vi "TSM SSC Fgen Pins to Sessions.vi"(0 "TSM context in":T3, 5 "Pins":string[](array[string]), 7 "Site Numbers":i32[](array[numeric]), 11 "error in":errorcluster) -> (4 "TSM FGEN":T1, 15 "error out":errorcluster)   [LabVIEW 2020]
doc: "Populates the TSM SSC Fgen cluster for the specified pin(s) and pin group(s)."
uses:
  <vilib>/NI_TestStand_SemiconductorModule/NI_TestStand_Semiconductor_Module.lvlibp/PinMap/General/SemiconductorModuleContext.ctl
  TSM SSC Fgen.ctl
  <vilib>/NI_TestStand_SemiconductorModule/NI_TestStand_Semiconductor_Module.lvlibp/PinMap/PinQueryContext/MultiplePinMultipleSessionQueryContext/MultiplePinMultipleSessionQueryContext.lvclass
  C:/Program Files/National Instruments/LabVIEW 2020/vi.lib/NI_TestStand_SemiconductorModule/NI_TestStand_Semiconductor_Module.lvlibp/PinMap/PinQueryContext/PinQueryContext.lvclass
  SSC Fgen.ctl
  <vilib>/NI_TestStand_SemiconductorModule/NI_TestStand_Semiconductor_Module.lvlibp/PinMap/FGEN/PinsToNIFGenSessions.vi
  <vilib>/NI_TestStand_SemiconductorModule/NI_TestStand_Semiconductor_Module.lvlibp
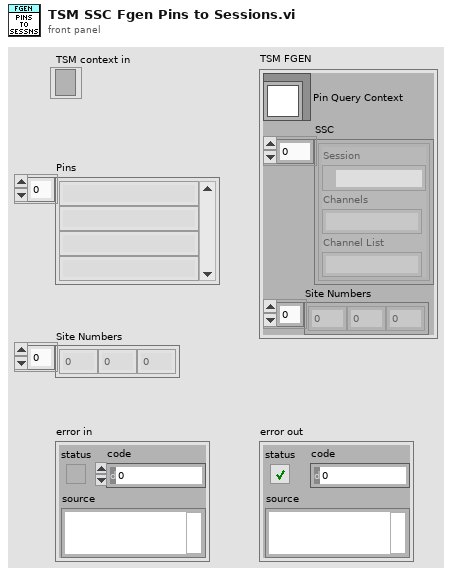
[diagram p1: front panel]
types:
  T1 = typedef "TSM SSC Fgen.ctl" = cluster{"Pin Query Context":refnum<class "MultiplePinMultipleSessionQueryContext.lvclass">, "SSC":T2[], "Site Numbers":i32[]}
  T2 = typedef "SSC Fgen.ctl" = cluster{"Session":refnum<k15>, "Channels":string, "Channel List":string}
  T3 = typedef "NI_TestStand_Semiconductor_Module.lvlibp/SemiconductorModuleContext.ctl" = refnum<k7>
  T4 = cluster{"Instrument Session":refnum<k15>, "Channel List":string, "spreadsheet string":string}[]
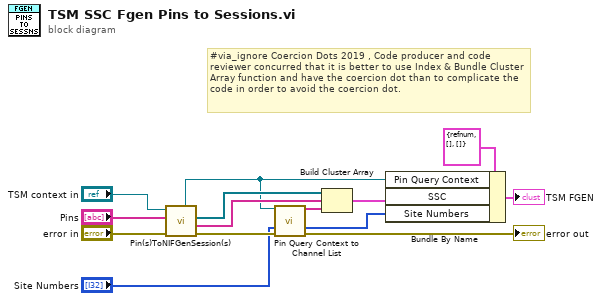
[diagram p0: block diagram]
diagram:
  # "#via_ignore Coercion Dots 2019 , Code producer and code reviewer concurred that it is better to use Index & Bundle Cluster Array function and have the coercion dot than to complicate the code in order to avoid the coercion dot."
  n1 = call-poly <vilib>:"Pin(s)ToNIFGenSession(s).vi"("error in (no error)"="error in", "Pins"="Pins", "Semiconductor Module Context"="TSM context in") -> ("error out"=w14:errorcluster, "Channel Lists"=w12:string[], "Instrument Sessions"=w13:refnum<k15>[], "Pin Query Context"=w10:refnum<class "MultiplePinMultipleSessionQueryContext.lvclass">)  [unwired: 4 in, 1 out]
  n2 = call "Pin Query Context to Channel List.vi"("Pin Query Context"=w10, "Site Numbers In"="Site Numbers", "error in"=w14) -> ("Per-Session Channel List"=w9:string[], "Site Numbers Out"=w1:i32[], "error out"=→"error out":errorcluster)  [unwired: 9 in, 1 out]
  n3 = Build Cluster Array(w13, w12, w9) -> (w11:T4)
  n4 = Bundle By Name(cluster=T1 {"Pin Query Context"=refnum, "SSC"=[], "Site Numbers"=[]} ("Fgen - Multiple Sessions Info"), "Pin Query Context"=w10, "SSC"=w11, "Site Numbers"=w1) -> (→"TSM FGEN":T1)
